vi "2D Array Subset.vi"() -> ()   [LabVIEW 2016]
panel:
  out "subarray":dbl[][](array[numeric])
  in  "length 2":i32
  in  "Row Index":i32
  in  "length":i32
  in  "Column Index":i32
  in  "array":dbl[][](array[numeric])
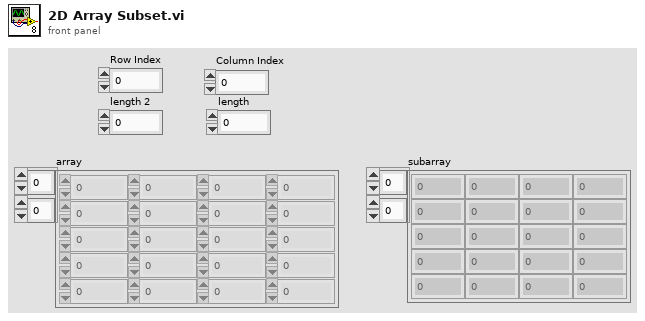
[diagram p1: front panel]
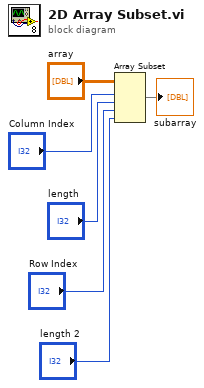
[diagram p0: block diagram]
diagram:
  n1 = Array Subset(array="array", index (row)="Column Index", length (row)="length", index (col)="Row Index", length (col)="length 2") -> (→"subarray":dbl[][])
